vi "Drive Get.vi"(1 "X All Power?":bool, 2 "Axis Y":dbl, 3 "Axis X":dbl) -> ()   [LabVIEW 2012]
uses:
  Drive Global Data.vi
panel:
  in  "Change Gear?":bool
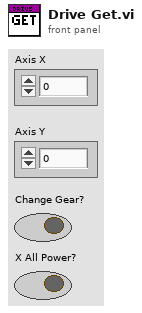
[diagram p1: front panel]
types:
  T1 = typedef "WPI_SolenoidValue.ctl" = enum16{"Off", "On", "Forward", "Reverse"}
  T2 = cluster{"Shifter?":bool, "Axisses":dbl[], "Shifter Value":T1}
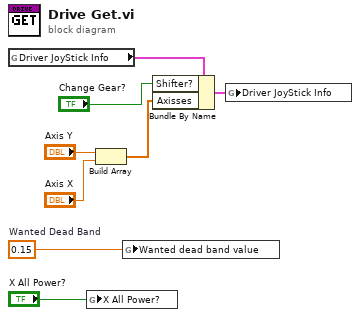
[diagram p0: block diagram]
diagram:
  w4 = 0.15  # Wanted Dead Band
  n1 = global read "Drive Global Data.vi" "Driver JoyStick Info"() -> (w8:T2)
  n2 = global write "Drive Global Data.vi" "X All Power?"("X All Power?") -> ()
  n3 = Build Array("Axis Y", "Axis X") -> (w7:dbl[])
  n4 = global write "Drive Global Data.vi" "Wanted dead band value"(w4) -> ()
  n5 = Bundle By Name(cluster=w8, "Shifter?"="Change Gear?", "Axisses"=w7) -> (w5:T2)
  n6 = global write "Drive Global Data.vi" "Driver JoyStick Info"(w5) -> ()
